vi "Aquisicao_Dados_IV.vi"() -> ()   [LabVIEW 2019]
uses:
  <vilib>/Utility/error.llb/DialogType.ctl
  <vilib>/Platform/TimedLoop/XDataNode/timing_clust.ctl
  <vilib>/Platform/TimedLoop/XDataNode/nitl_modes.ctl
  <vilib>/Platform/TimedLoop/XDataNode/wakeup.ctl
  <vilib>/DAQmx/write.llb/DAQmx Write (Analog 1D DBL NChan 1Samp).vi
  <vilib>/DAQmx/read.llb/DAQmx Read (Analog 1D DBL NChan 1Samp).vi
  <vilib>/DAQmx/create/channels.llb/DAQmx Create Channel (AI-Voltage-Basic).vi
  <vilib>/DAQmx/configure/timing.llb/DAQmx Timing (Sample Clock).vi
  <vilib>/DAQmx/create/channels.llb/DAQmx Create Channel (AO-Voltage-Basic).vi
  <vilib>/DAQmx/miscellaneous.llb/DAQmx Fill In Error Info.vi
  <vilib>/platform/TimedLoop/XDataNode/XDataNode.xnode
  <vilib>/Platform/TimedLoop/XDataNode/XDNodeRunTimeDep.lvlib
panel:
  in  "SIMULACAO PRESSAO":dbl(slide) scale=0.0..200.0
  in  "Pausa inspiração (s)":dbl=1.0
  in  "Frequência respiratória (rpm)":dbl=6.0
  in  "Início?":bool
  in  "Next State":T1(ring)=enum."Expiração descendo pressão"
  out "Expiração início":u32
  out "Tempo pressão constante início":u32
  out "Pa, Pb e Ps":dbl[][](graph)
  in  "Pressão de referencia [cmH2O]":dbl(slide) scale=0.0..200.0
  in  "?":bool
  in  "Salvar Dados? 3":bool
  out "Posição e Referência":dbl[][](graph)
  out "Segundos":u32
  # "Passo a passo:\n\n1 - Executar o VI;\n2 - Decidir se deseja salvar ou não os dados, caso deseje, pressione o botão \"Salvar dados\";\n3 - Decidir se deseja controlar o sistema em malha aberta ou fechada, caso deseje malha fechada, pressione o botão \"Malha Fechada\";\n3.1 - Em malha fechada, aplique os ganhos do controlador PID na janela PID Gains. Ajuste a referência no botão de deslizamneto. \n        Caso seja necessário, resete o integrador pelo botão \"Resetar PID\";\n3.2 - Em malha aberta, selecione o valor da tensão a ser aplicada na válvula prporcional (-10 a 10 V)\n4 - Ao final, pressione o botão \"STOP\"\n5 - Se desejar visualizar os dados, os mesmo foram salvos em um arquivo .tdms na pasta XXXX, e o nome dele segue o seguinte fomrato \n      \"Daodos_Ano_Mês_Dia_Hora_Segundo\". Para visualizar, utilize o programa SuperViewer."
  # "Controle"
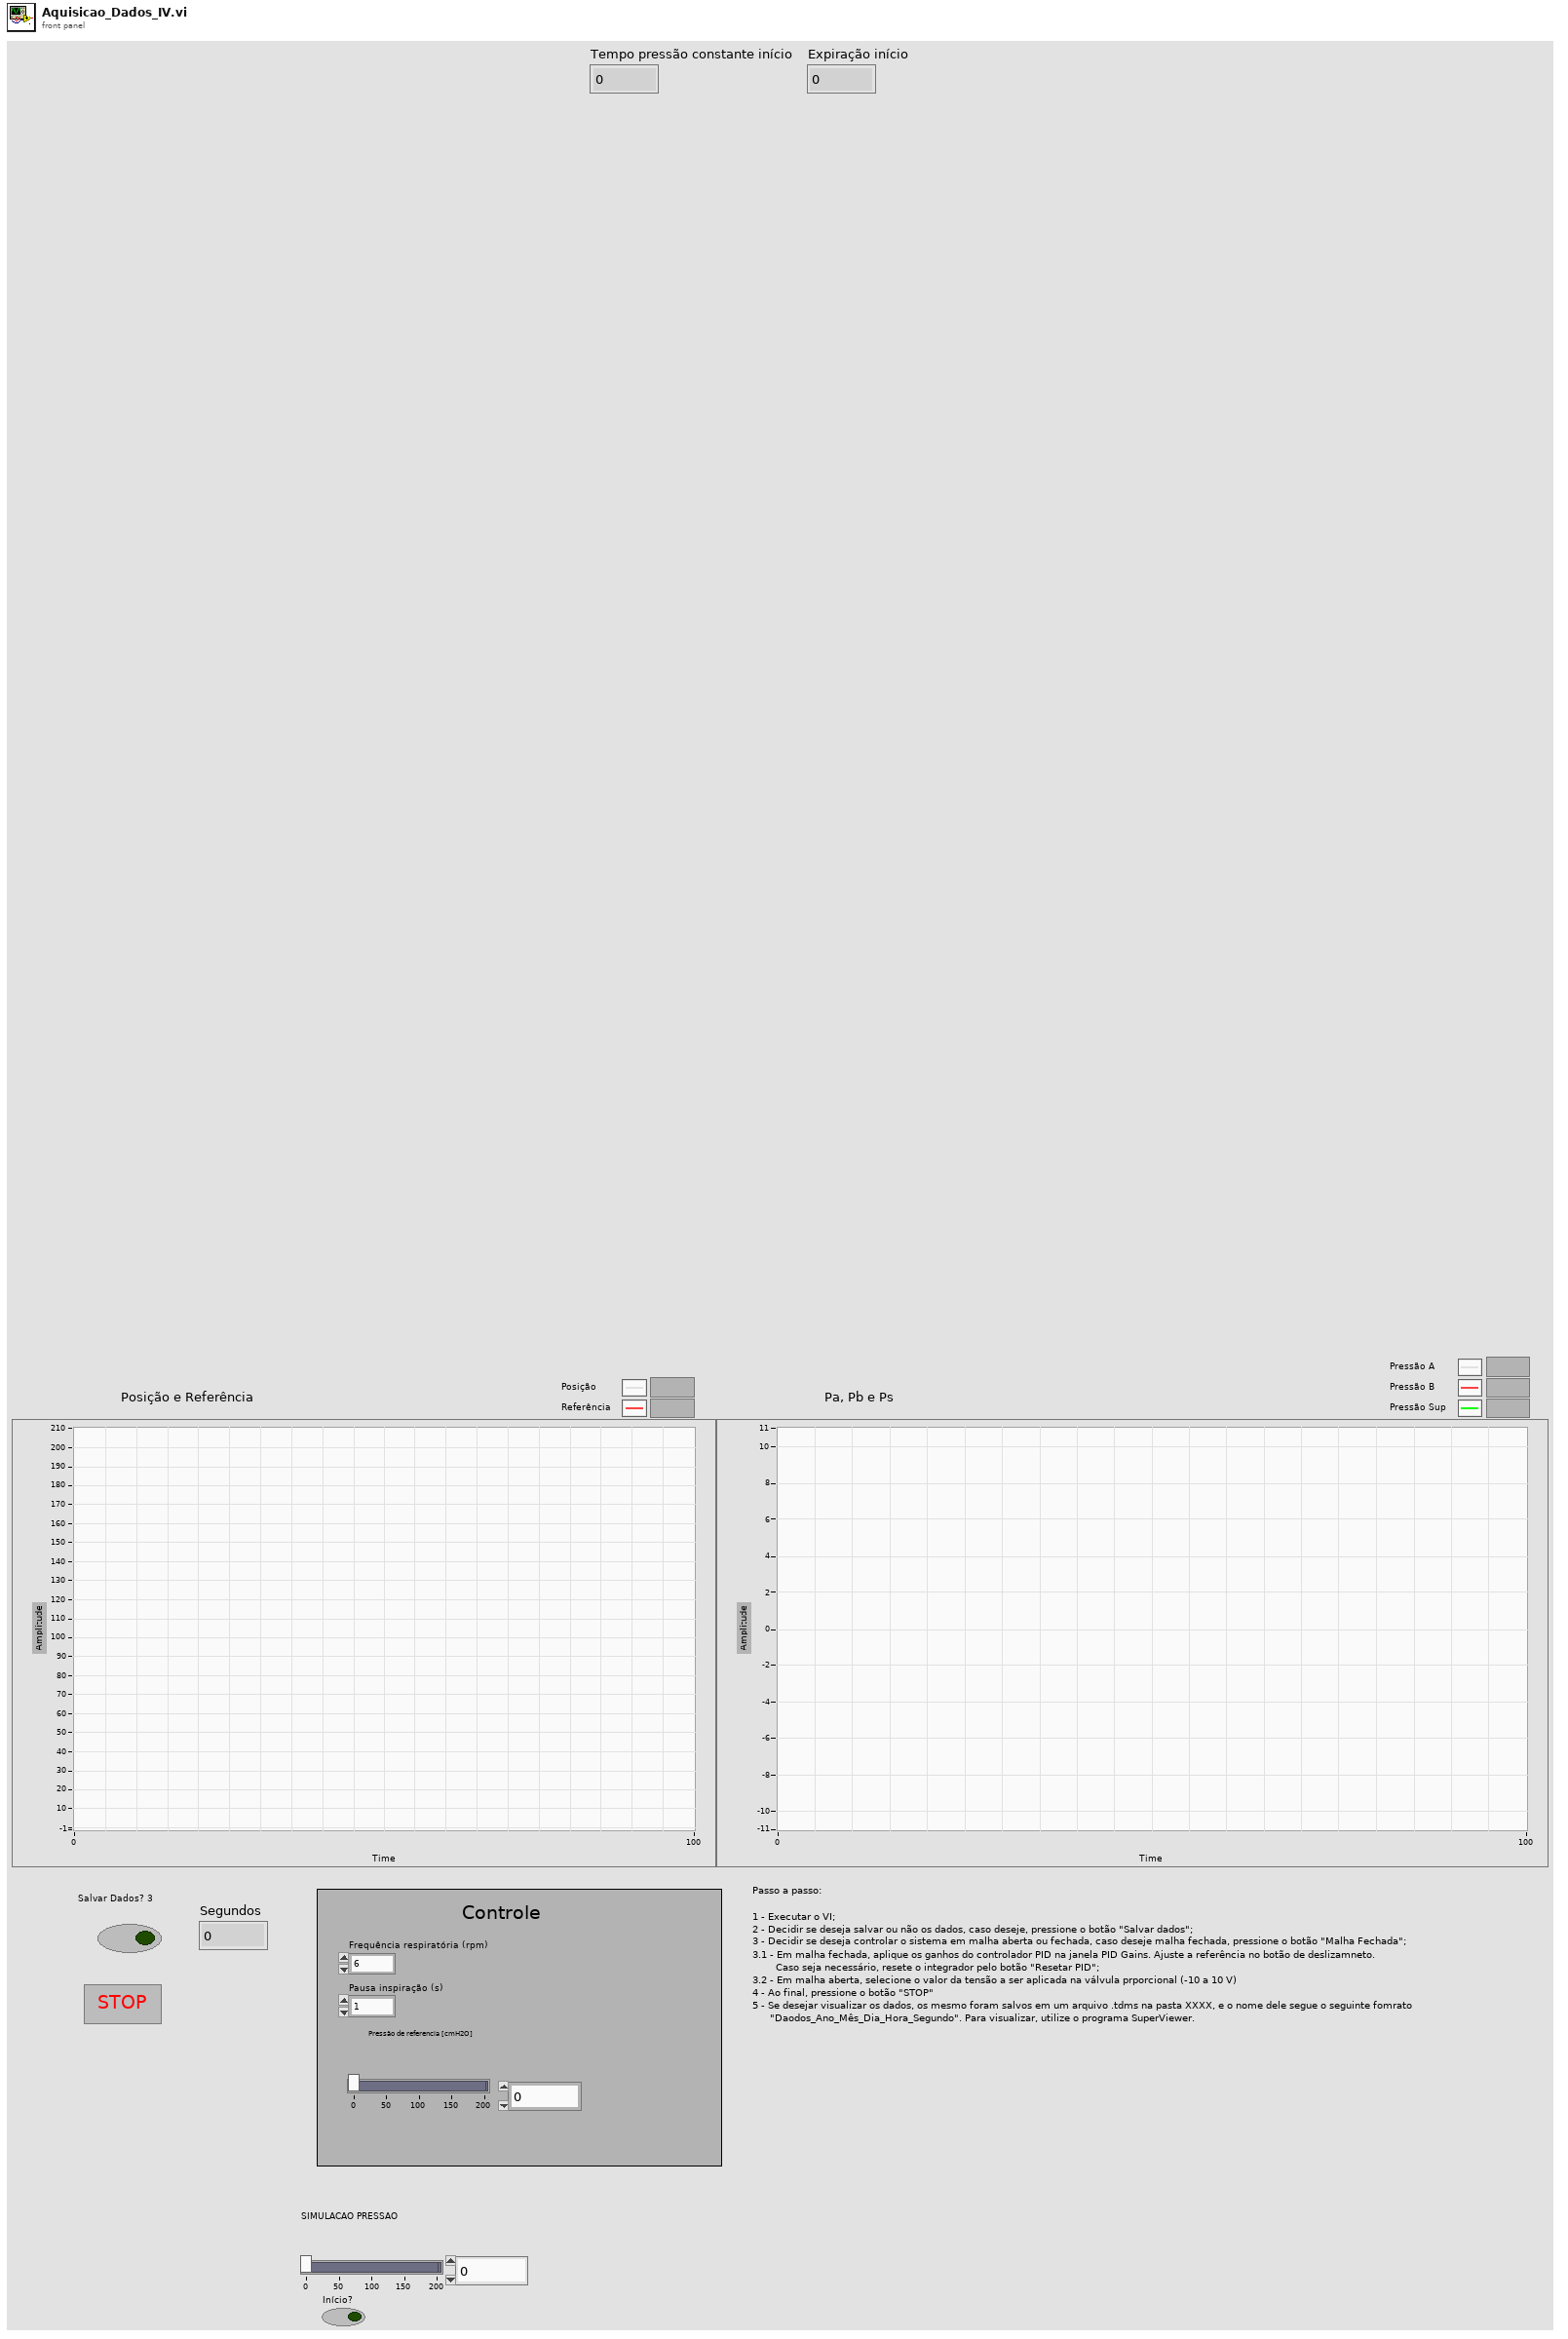
[diagram p1: front panel]
types:
  T1 = enum16{"Inspiração: subindo pressão", "Inspiração: pressão constante", "Expiração descendo pressão"}
  T2 = enum16{"open", "open or create", "create or replace", "create", "open (read-only)"}
  T3 = typedef "DialogType.ctl" = u16
  T4 = typedef "XDNodeRunTimeDep.lvlib/timing_clust.ctl" = cluster{"Expected End [f-1]":u64, "Actual End [f-1]":u64, "Finished Late? [f-1]":bool, "Expected End [i-1]":u64, "Actual End [i-1]":u64, "Finished Late? [i-1]":bool, "Expected Start [i]":u64, "Actual Start [i]":u64, "Expected Start [f]":u64, "Actual Start [f]":u64, "Source Name":string, "Structure Name":string, "Period":i64, "Deadline":i64, "Offset":i64, "Start":i64, "Priority":i32, "Timeout":i32, "Mode":T5, "Wakeup Reason":T6, "Error":errorcluster, "Source Type":string, "Secondary Source Type":string, "Global End Time":u64, "Global Start Time":u64, "Frame Duration":u64, "Iteration Duration":u64, "Assigned CPU":i32, "I/O Scan Engine Mode":u32}
  T5 = typedef "XDNodeRunTimeDep.lvlib/nitl_modes.ctl" = enum32{"No Change", "Process missed periods, maintain original phase", "Discard missed periods, maintain original phase", "Process missed periods, ignore original phase", "Discard missed periods, ignore original phase"}
  T6 = typedef "XDNodeRunTimeDep.lvlib/wakeup.ctl" = enum32{"Normal", "Aborted", "Asynchronous wakeup", "Timing source error", "Timed loop error", "Timeout"}
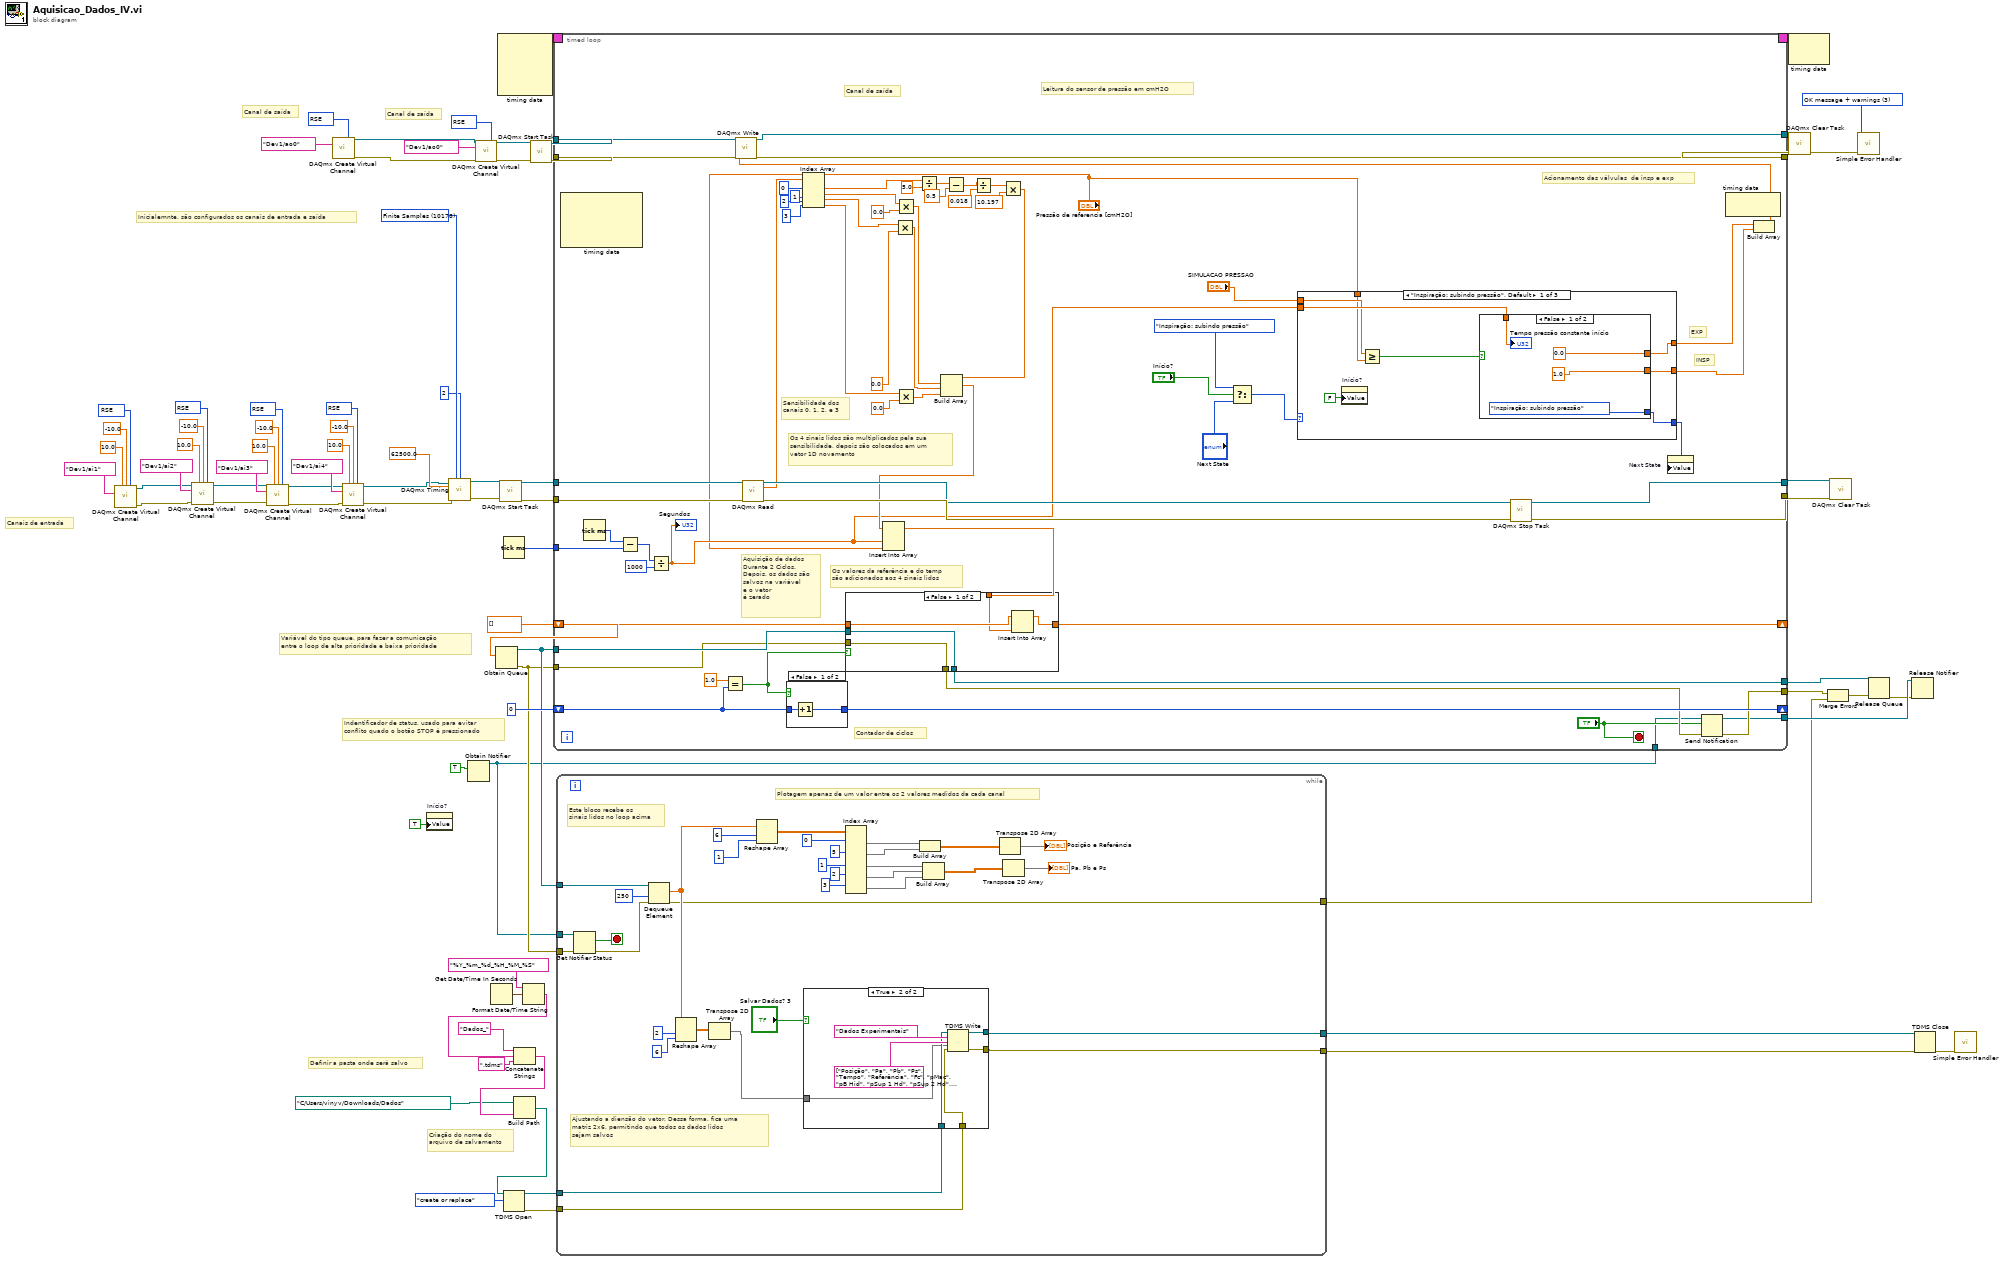
[diagram p0: block diagram]
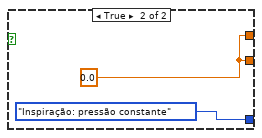
[diagram p2: hidden frame]
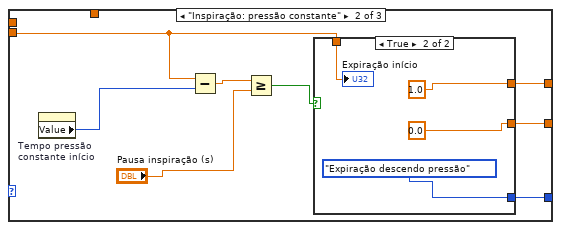
[diagram p3: hidden frame]
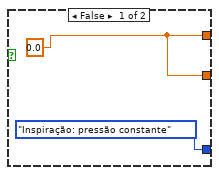
[diagram p4: hidden frame]
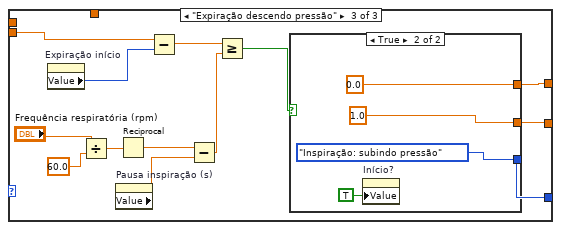
[diagram p5: hidden frame]
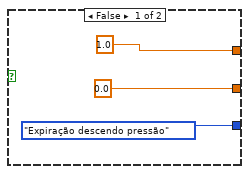
[diagram p6: hidden frame]
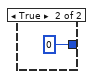
[diagram p7: hidden frame]
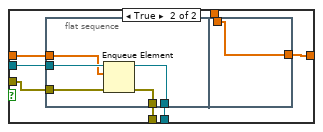
[diagram p8: hidden frame]
diagram:
  w5 = 10083 items=["Default"=-1, "RSE"=10083, "NRSE"=10078, "Differential"=10106, "Pseudodifferential"=12529] ("input terminal configuration")
  w39 = T3 3 items=["no dialog", "OK message", "continue or stop message", "OK message + warnings", "continue/stop + warnings"] ("type of dialog (OK msg:1)")
  w40 = 10083 items=["Default"=-1, "RSE"=10083, "NRSE"=10078, "Differential"=10106, "Pseudodifferential"=12529] ("input terminal configuration")
  w58 = 10083 items=["Default"=-1, "RSE"=10083, "NRSE"=10078, "Differential"=10106, "Pseudodifferential"=12529] ("input terminal configuration")
  w62 = 10083 items=["Default"=-1, "RSE"=10083, "NRSE"=10078, "Differential"=10106, "Pseudodifferential"=12529] ("input terminal configuration")
  w66 = 10083 items=["Default"=-1, "RSE"=10083, "NRSE"=10078, "Differential"=10106, "Pseudodifferential"=12529] ("input terminal configuration")
  w41 = dbl[] []
  w72 = 10178 items=["Finite Samples"=10178, "Continuous Samples"=10123, "Hardware Timed Single Point"=12522] ("sample mode")
  w75 = 10083 items=["Default"=-1, "RSE"=10083, "NRSE"=10078, "Differential"=10106, "Pseudodifferential"=12529] ("input terminal configuration")
  # "Canal de saída"
  # "Definir a pasta onde será salvo"
  # "Indentificador de status, usado para evitar \nconflito quado o botão STOP é pressionado"
  # "Variável do tipo queue, para fazer a comunicação \nentre o loop de alta prioridade e baixa prioridade"
  # "Canais de entrada"
  # "Canal de saída"
  # "Inicialemnte, são configurados os canais de entrada e saída"
  # "Criação do nome do\narquivo de salvamento"
  n1 = call-poly <vilib>:"DAQmx Create Virtual Channel.vi"("maximum value"=10.0, "minimum value"=-10.0, "input terminal configuration"=w58, "physical channels"=tag "Dev1/ai1") -> ("task out"=w54:refnum<k21>, "error out"=w53:errorcluster)  [unwired: 10 in]
  n2 = call-poly <vilib>:"DAQmx Create Virtual Channel.vi"("task in"=w54, "maximum value"=10.0, "minimum value"=-10.0, "input terminal configuration"=w75, "physical channels"=tag "Dev1/ai2", "error in"=w53) -> ("task out"=w52:refnum<k21>, "error out"=w51:errorcluster)  [unwired: 8 in]
  n3 = call-poly <vilib>:"DAQmx Create Virtual Channel.vi"("task in"=w52, "maximum value"=10.0, "minimum value"=-10.0, "input terminal configuration"=w66, "physical channels"=tag "Dev1/ai3", "error in"=w51) -> ("task out"=w50:refnum<k21>, "error out"=w49:errorcluster)  [unwired: 8 in]
  n4 = call-poly <vilib>:"DAQmx Create Virtual Channel.vi"("output terminal configuration"=w5, "physical channels"=tag "Dev1/ao0") -> ("task out"=w3:refnum<k21>, "error out"=w2:errorcluster)  [unwired: 12 in]
  n5 = call-poly <vilib>:"DAQmx Create Virtual Channel.vi"("task in"=w50, "maximum value"=10.0, "minimum value"=-10.0, "input terminal configuration"=w62, "physical channels"=tag "Dev1/ai4", "error in"=w49) -> ("task out"=w48:refnum<k21>, "error out"=w47:errorcluster)  [unwired: 8 in]
  n6 = property on="Início?" class="Bool (strict)"("Value"=TRUE ("Início?")) -> ()  [unwired: 2 in, 2 out]
  n7 = call-poly <vilib>:"DAQmx Timing.vi"("task/channels in"=w48, "sample mode"=w72, "samples per channel"=2, "rate"=62500.0, "error in"=w47) -> ("task out"=w71:refnum<k21>, "error out"=w70:errorcluster)  [unwired: 9 in]
  n8 = Obtain Notifier(notification data type=TRUE) -> (notifier out=w10:refnum<notifier>)  [unwired: 3 in, 2 out]
  n9 = call-poly <vilib>:"DAQmx Create Virtual Channel.vi"("task in"=w3, "output terminal configuration"=w40, "physical channels"=tag "Dev1/ao0", "error in"=w2) -> ("task out"=w36:refnum<k21>, "error out"=w35:errorcluster)  [unwired: 10 in]
  n10 = Get Date/Time In Seconds() -> (seconds since 1Jan1904=w25:timestamp)
  n11 = Obtain Queue(element data type=w41) -> (queue out=w29:refnum<queue>, error out=w12:errorcluster)  [unwired: 4 in, 1 out]
  n12 = node-c288() -> (w77:T4)  [unwired: 4 in]
  n13 = call <vilib>:"DAQmx Start Task.vi"("task/channels in"=w71, "error in"=w70) -> ("task out"=w46:refnum<k21>, "error out"=w45:errorcluster)  [unwired: 12 in]
  n14 = Tick Count (ms)() -> (millisecond timer value=w30:u32)
  n15 = Format Date/Time String(time format string (%c)="%Y_%m_%d_%H_%M_%S", seconds (now)=w25) -> (date/time string=w26:string)  [unwired: 1 in]
  n16 = Concatenate Strings("Dados_" ("name or relative path"), w26, ".tdms" ("string")) -> (w27:string)
  n17 = Build Path(base path=path "C:/Users/vinyv/Downloads/Dados", name or relative path=w27) -> (appended path=w20:path)
  n18 = TDMS Open(10:T2."create or replace" ("operation (0:open)"), 11:w20) -> (0:w18:errorcluster, 3:w19:refnum<k34>)  [unwired: 5 in]
  n19 = call <vilib>:"DAQmx Start Task.vi"("task/channels in"=w36, "error in"=w35) -> ("task out"=w34:refnum<k21>, "error out"=w33:errorcluster)  [unwired: 12 in]
  n20 = timed-loop {
    timing: w77 -> [_]
    timing-out: [_] -> w76
    tunnel: w46 -> [w141]
    tunnel: w45 -> [w140]
    tunnel: [w121] -> w44
    tunnel: [w120] -> w43
    shift-right: [w138] -> _
    shift-left: 0 -> [w137]
    shift-right: [w119] -> _
    shift-left: w41 -> [w135]
    tunnel: w29 -> [w134]
    tunnel: w12 -> [w133]
    tunnel: [w132] -> w14
    tunnel: [w101] -> w7
    tunnel: w34 -> [w131]
    tunnel: w33 -> [w130]
    tunnel: [w129] -> w32
    tunnel: [w128] -> w31
    tunnel: w30 -> [w126]
    tunnel: [w99] -> w13
    tunnel: w10 -> [w98]
    stop <- "?" stop-if-true
    # "INSP"
    # "EXP"
    # "Acionamento das válvulas  de insp e exp"
    # "Leitura do sensor de pressão em cmH2O"
    # "Os valores da referência e do temp \nsão adicionados aos 4 sinais lidos"
    # "Os 4 sinais lidos são multiplicados pela sua\nsensibilidade, depois são colocados em um \nvetor 1D novamento"
    # "Canal de saída"
    # "Sensibilidade dos \ncanais 0, 1, 2, e 3"
    # "Contador de ciclos"
    # "Aquisição de dados\nDurante 2 Ciclos. \nDepois, os dados são\nsalvos na variável\ne o vetor\né zerado"
    n21 = node-c288() -> ()  [unwired: 1 in, 4 out]
    n22 = Tick Count (ms)() -> (millisecond timer value=w127:u32)
    n23 = Subtract(x=w127, y=w126) -> (x-y=w125:u32)
    n24 = Divide(x=w125, y=u32 1000) -> (x/y=w83:dbl)
    "Segundos" <- w83
    n25 = Equal?(x=1.0, y=w137) -> (x = y?=w136:bool)
    n26 = call-poly <vilib>:"DAQmx Read.vi"("task/channels in"=w141, "error in"=w140) -> ("task out"=w122:refnum<k21>, "data"=w117:dbl[], "error out"=w123:errorcluster)  [unwired: 11 in]
    n27 = case shown="False" w136 {
      tunnel: [w191 0] -> w138
      tunnel: w137 -> [w190 _]
      frame False {
        n28 = Increment(x=w190) -> (x+1=w191:i32)
      }
      frame True {
      }
    }
    n29 = Index Array(array=w117, index #1=0 ("index"), index #2=1 ("index"), index #3=2 ("index"), index #4=3 ("index")) -> (element #1=w96:dbl, element #2=w109:dbl, element #3=w108:dbl, element #4=w107:dbl)
    n30 = Multiply(x=w108, y=0.0) -> (x*y=w105:dbl)
    n31 = Multiply(x=w109, y=0.0) -> (x*y=w106:dbl)
    n32 = Multiply(x=w107, y=0.0) -> (x*y=w104:dbl)
    n33 = Divide(x=w96, y=5.0 ("x")) -> (x/y=w94:dbl)
    n34 = Subtract(x=w94, y=0.5) -> (x-y=w92:dbl)
    n35 = Divide(x=w92, y=0.018) -> (x/y=w90:dbl)
    n36 = Multiply(x=w90, y=10.197) -> (x*y=w82:dbl)
    n37 = Build Array(w82, w106, w105, w104) -> (w103:dbl[])
    n38 = Insert Into Array(array=w103, new element #1=w83, new element #2="Pressão de referencia [cmH2O]") -> (w118:dbl[])  [unwired: 1 in]
    n39 = case shown="False" w136 {
      tunnel: [w197 w204] -> w119
      tunnel: w135 -> [w196 w199]
      tunnel: w134 -> [w195 w203]
      tunnel: w133 -> [w194 w202]
      tunnel: [w195 w201] -> w132
      tunnel: [w194 w200] -> w102
      tunnel: w118 -> [w193 w198]
      frame False {
        n40 = Insert Into Array(array=w196, new element=w193) -> (w197:dbl[])  [unwired: 1 in]
      }
      frame True {
        n41 = flat-sequence {
          tunnel: w203 -> [w209]
          tunnel: w202 -> [w208]
          tunnel: [w207] -> w201
          tunnel: [w206] -> w200
          tunnel: w199 -> [w205]
          tunnel: [w210] -> w204
          tunnel: w198 -> [w210]
          frame #0 {
            n42 = Enqueue Element(queue=w209, element=w205, error in (no error)=w208) -> (queue out=w207:refnum<queue>, error out=w206:errorcluster)  [unwired: 1 in, 1 out]
          }
          frame #1 {
          }
        }
      }
    }
    n43 = Select(t=T1."Inspiração: subindo pressão", s="Início?", f="Next State") -> (s? t:f=w85:T1)
    n44 = case shown="\"Inspiração: subindo pressão\", Default" w85 {
      tunnel: [w148 w160 w173] -> w84
      tunnel: w83 -> [w147 w159 w178]
      tunnel: "SIMULACAO PRESSAO" -> [w146 _ _]
      tunnel: "Pressão de referencia [cmH2O]" -> [w145 _ _]
      tunnel: [w143 w157 w171] -> w80
      tunnel: [w142 w156 w170] -> w79
      frame "Inspiração: subindo pressão", Default {
        n45 = property on="Início?" class="Bool (strict)"("Value"=FALSE ("Início?")) -> ()  [unwired: 2 in, 2 out]
        n46 = Greater Or Equal?(x=w146, y=w145) -> (x >= y?=w149:bool)
        n47 = case shown="False" w149 {
          tunnel: [T1."Inspiração: subindo pressão" T1."Inspiração: pressão constante"] -> w148
          tunnel: w147 -> [w152 _]
          tunnel: [0.0 ("Válvula expiração") w154] -> w143
          tunnel: [1.0 ("Válvula Inspiração") w154] -> w142
          frame False {
            "Tempo pressão constante início" <- w152
          }
          frame True {
            w154 = 0.0 ("Válvula expiração")
          }
        }
      }
      frame "Inspiração: pressão constante" {
        n48 = property on="Tempo pressão constante início" class="DigNum (strict)"() -> ("Value"=w163:u32)  [unwired: 2 in, 2 out]
        n49 = Subtract(x=w159, y=w163) -> (x-y=w162:dbl)
        n50 = Greater Or Equal?(x=w162, y="Pausa inspiração (s)") -> (x >= y?=w161:bool)
        n51 = case shown="True" w161 {
          tunnel: [T1."Inspiração: pressão constante" T1."Expiração descendo pressão"] -> w160
          tunnel: w159 -> [_ w168]
          tunnel: [w164 1.0 ("Válvula expiração")] -> w157
          tunnel: [w164 0.0 ("Válvula Inspiração")] -> w156
          frame False {
            w164 = 0.0 ("Válvula Inspiração")
          }
          frame True {
            "Expiração início" <- w168
          }
        }
      }
      frame "Expiração descendo pressão" {
        n52 = property on="Expiração início" class="DigNum (strict)"() -> ("Value"=w177:u32)  [unwired: 2 in, 2 out]
        n53 = Divide(x="Frequência respiratória (rpm)", y=60.0) -> (x/y=w180:dbl)
        n54 = property on="Pausa inspiração (s)" class="DigNum (strict)"() -> ("Value"=w179:dbl)  [unwired: 2 in, 2 out]
        n55 = Reciprocal(x=w180) -> (1/x=w182:dbl)
        n56 = Subtract(x=w178, y=w177) -> (x-y=w176:dbl)
        n57 = Subtract(x=w182, y=w179) -> (x-y=w175:dbl)
        n58 = Greater Or Equal?(x=w176, y=w175) -> (x >= y?=w174:bool)
        n59 = case shown="True" w174 {
          tunnel: [T1."Expiração descendo pressão" T1."Inspiração: subindo pressão"] -> w173
          tunnel: [1.0 ("Válvula expiração") 0.0 ("Válvula expiração")] -> w171
          tunnel: [0.0 ("Válvula Inspiração") 1.0 ("Válvula Inspiração")] -> w170
          frame False {
          }
          frame True {
            n60 = property on="Início?" class="Bool (strict)"("Value"=TRUE ("Início?")) -> ()  [unwired: 2 in, 2 out]
          }
        }
      }
    }
    n61 = call <vilib>:"DAQmx Stop Task.vi"("task/channels in"=w122, "error in"=w123) -> ("task out"=w121:refnum<k21>, "error out"=w120:errorcluster)  [unwired: 12 in]
    n62 = property on="Next State" class="Enum (strict)"("Value"=w84) -> ()  [unwired: 2 in, 2 out]
    n63 = Send Notification(notification="?", notifier=w98, error in (no error)=w102) -> (notifier out=w99:refnum<notifier>, error out=w101:errorcluster)
    n64 = node-c288() -> ()  [unwired: 1 in, 1 out]
    n65 = Build Array(w80, w79) -> (w97:dbl[])
    n66 = call-poly <vilib>:"DAQmx Write.vi"("task/channels in"=w131, "data"=w97, "error in"=w130) -> ("task out"=w129:refnum<k21>, "error out"=w128:errorcluster)  [unwired: 10 in, 1 out]
  }
  n67 = while {
    tunnel: w29 -> [w235]
    tunnel: w19 -> [w233]
    tunnel: w18 -> [w232]
    tunnel: [w231] -> w16
    tunnel: [w230] -> w15
    tunnel: w10 -> [w218]
    tunnel: w12 -> [w217]
    tunnel: [w214] -> w8
    stop <- w215 stop-if-true
    # "Este bloco recebe os \nsinais lidos no loop acima"
    # "Ajustando a diensão do vetor. Dessa forma, fica uma \nmatriz 2x6, permitindo que todos os dados lidos \nsejam salvos"
    # "Plotagem apenas de um valor entre os 2 valores medidos da cada canal"
    n68 = Get Notifier Status(notifier=w218, error in (no error)=w217) -> (current notification=w215:bool, error out=w216:errorcluster)  [unwired: 3 out]
    n69 = Dequeue Element(queue=w235, timeout in ms (-1)=250, error in (no error)=w216) -> (element=w226:dbl[], error out=w214:errorcluster)  [unwired: 2 out]
    n70 = Reshape Array(w226, 2 ("dimension size"), 6 ("dimension size")) -> (w228:dbl[][])
    n71 = Transpose 2D Array(2D array=w228) -> (transposed array=w227:dbl[][])
    n72 = Reshape Array(w226, 6 ("dimension size"), 1 ("dimension size")) -> (w239:dbl[][])
    n73 = case shown="True" "Salvar Dados? 3" {
      tunnel: w233 -> [w247 w253]
      tunnel: w232 -> [w248 w252]
      tunnel: [w247 w251] -> w231
      tunnel: [w248 w250] -> w230
      tunnel: w227 -> [_ w249]
      frame False {
      }
      frame True {
        n74 = TDMS Write(0:w253, 5:"Dados Experimentais" ("group name in (Untitled)"), 7:string[] ["Posição", "Pa", "Pb", "Ps", "Tempo", "Referência", "Fc", "pMac", "pB Hid", "pSup 1 Hd", "pSup 2 Hd", "pA Pn", "pB Pn", "Enc", "Tempo", "Ta", "Tb", "Ts", "Velocidade"] ("channel name(s) in (Untitled)"), 9:w249, 11:w252) -> (4:w251:refnum<k34>, 15:w250:errorcluster)  [unwired: 1 in, 2 out]
      }
    }
    n75 = Index Array(array=w239, index (row) #1=0 ("index (row)"), index (row) #2=5 ("index (row)"), index (row) #3=1 ("index (row)"), index (row) #4=2 ("index (row)"), index (row) #5=3 ("index (row)")) -> (element #1=w236:dbl[], element #2=w240:dbl[], element #3=w221:dbl[], element #4=w220:dbl[], element #5=w219:dbl[])  [unwired: 5 in]
    n76 = Build Array(w236, w240) -> (w238:dbl[][])
    n77 = Build Array(w221, w220, w219) -> (w225:dbl[][])
    n78 = Transpose 2D Array(2D array=w238) -> (transposed array=→"Posição e Referência":dbl[][])
    n79 = Transpose 2D Array(2D array=w225) -> (transposed array=→"Pa, Pb e Ps":dbl[][])
  }
  n80 = node-c288(w76) -> ()  [unwired: 1 out]
  n81 = call <vilib>:"DAQmx Clear Task.vi"("task in"=w32, "error in"=w31) -> ("error out"=w38:errorcluster)  [unwired: 13 in]
  n82 = Merge Errors(w7, w8) -> (w6:errorcluster)
  n83 = call <vilib>:"DAQmx Clear Task.vi"("task in"=w44, "error in"=w43) -> ()  [unwired: 13 in, 1 out]
  n84 = call <vilib>:"Simple Error Handler.vi"("type of dialog (OK msg:1)"=w39, "error in (no error)"=w38) -> ()  [unwired: 3 in, 5 out]
  n85 = Release Queue(queue=w14, error in (no error)=w6) -> (error out=w9:errorcluster)  [unwired: 1 in, 2 out]
  n86 = Release Notifier(notifier=w13, error in (no error)=w9) -> ()  [unwired: 1 in, 3 out]
  n87 = TDMS Close(8:w15, 11:w16) -> (0:w17:errorcluster)  [unwired: 1 out]
  n88 = call <vilib>:"Simple Error Handler.vi"("error in (no error)"=w17) -> ()  [unwired: 4 in, 5 out]
